vi "motor_stage.vi"() -> ()   [LabVIEW 2016]
uses:
  <vilib>/Instr/_visa.llb/VISA Configure Serial Port (Instr).vi
panel:
  in  "stop":bool
  in  "Boolean":bool
  in  "String":string
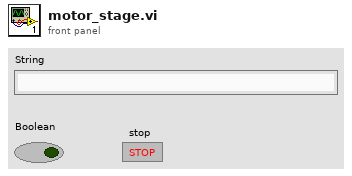
[diagram p1: front panel]
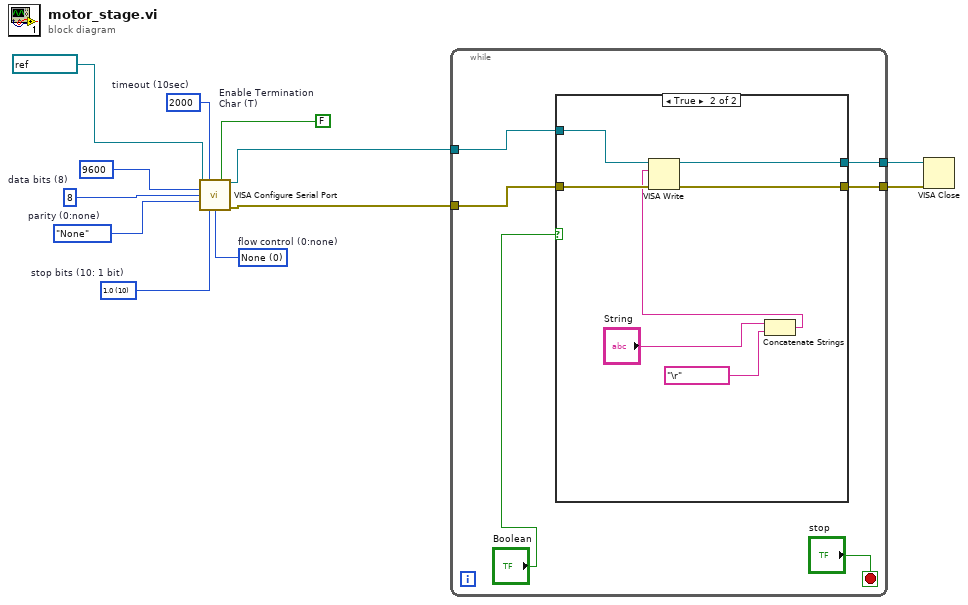
[diagram p0: block diagram]
diagram:
  w4 = u16 0 items=["None", "XON/XOFF", "RTS/CTS", "XON/XOFF & RTS/CTS", "DTR/DSR", "XON/XOFF & DTR/DSR"]  # flow control (0:none)
  w5 = u16 10 items=["1.0"=10, "1.5"=15, "2.0"=20]  # stop bits (10: 1 bit)
  w8 = FALSE  # Enable Termination Char (T)
  w9 = u32 2000  # timeout (10sec)
  w10 = enum16{"None", "Odd", "Even", "Mark", "Space"}."None"  # parity (0:none)
  w11 = u16 8  # data bits (8)
  n1 = call-poly "VISA Configure Serial Port"("VISA resource name"=refnum<visa-resource-name> "COM4", "timeout (10sec)"=w9, "Enable Termination\nChar (T)"=w8, "baud rate (9600)"=u32 9600, "data bits (8)"=w11, "parity (0:none)"=w10, "stop bits (10: 1 bit)"=w5, "flow control (0:none)"=w4) -> ("VISA resource name out"=w7:refnum<visa-resource-name>, "error out"=w6:errorcluster)  [unwired: 6 in]
  n2 = while {
    tunnel: w7 -> [w18]
    tunnel: w6 -> [w17]
    tunnel: [w14] -> w2
    tunnel: [w13] -> w1
    stop <- "stop" stop-if-true
    n3 = case shown="True" "Boolean" {
      tunnel: w18 -> [w20 w27]
      tunnel: w17 -> [w19 w26]
      tunnel: [w19 w23] -> w14
      tunnel: [w20 w22] -> w13
      frame False {
      }
      frame True {
        n4 = Concatenate Strings("String", "\r" ("write buffer")) -> (w24:string)
        n5 = VISA Write(VISA resource name=w27, write buffer=w24, error in (no error)=w26) -> (VISA resource name out=w22:refnum<visa-resource-name>, error out=w23:errorcluster)  [unwired: 1 out]
      }
    }
  }
  n6 = VISA Close(VISA resource name=w1, error in (no error)=w2) -> ()  [unwired: 1 out]
